vi "Add.vi"(0 "object in":refnum<class "Node.lvclass">, 2 "Value":dbl, 5 "Error In":errorcluster) -> (14 "object out":refnum<class "Node.lvclass">, 19 "Error Out":errorcluster)   [LabVIEW 2024, in "Node.lvclass"]
uses:
  Node.lvclass
  Node.lvclass/Node.ctl
  Element_interface/Element.lvclass
panel:
  # "Connector Pane"
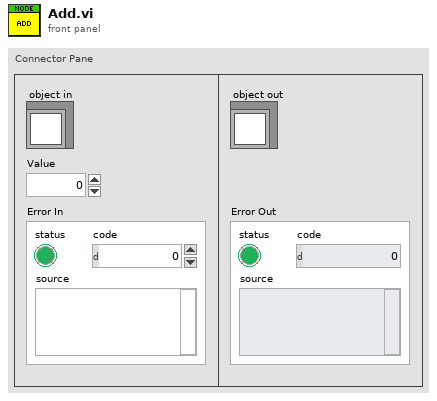
[diagram p1: front panel]
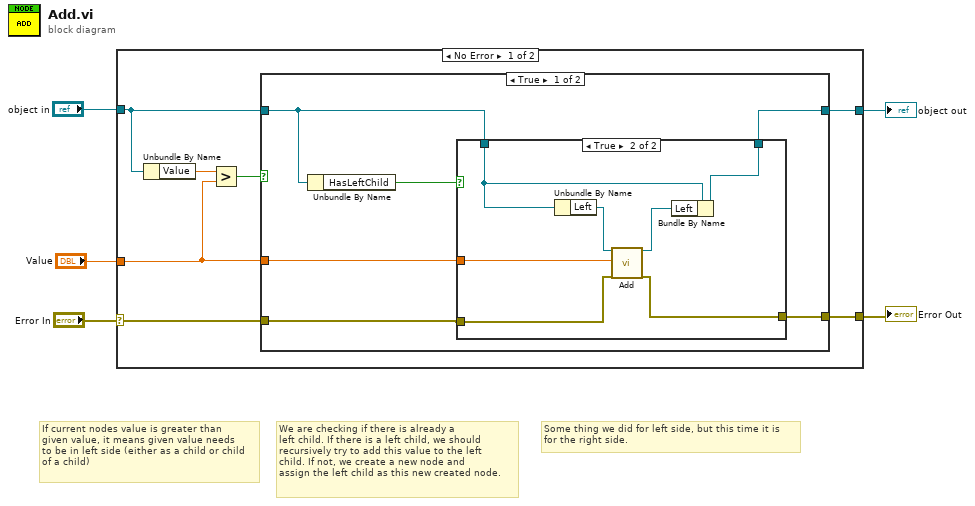
[diagram p0: block diagram]
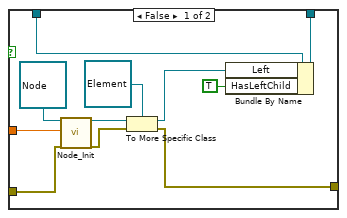
[diagram p2: hidden frame]
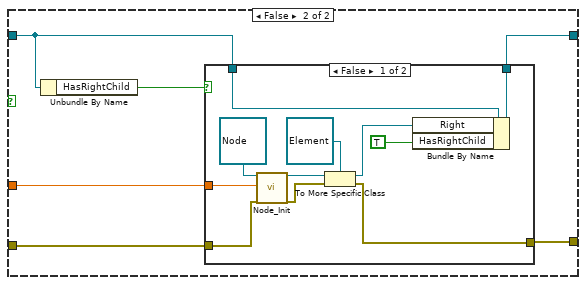
[diagram p3: hidden frame]
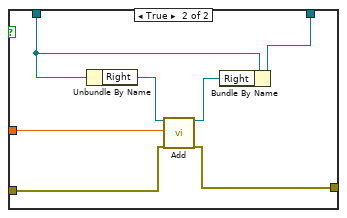
[diagram p4: hidden frame]
diagram:
  # "Some thing we did for left side, but this time it is\nfor the right side."
  # "We are checking if there is already a \nleft child. If there is a left child, we should\nrecursively try to add this value to the left\nchild. If not, we create a new node and \nassign the left child as this new created node."
  # "If current nodes value is greater than\ngiven value, it means given value needs\nto be in left side (either as a child or child\nof a child)"
  n1 = case shown="No Error" "Error In" {
    selector: "Error In" -> [w8 w62]
    tunnel: [w7 w62] -> w4
    tunnel: [w10 w61] -> w2
    tunnel: "object in" -> [w11 w61]
    tunnel: "Value" -> [w9 _]
    frame No Error {
      n2 = Unbundle By Name(w11) -> ("Value"=w6:dbl)
      n3 = Greater?(x=w6, y=w9) -> (0:w12:bool)
      n4 = case shown="True" w12 {
        tunnel: w11 -> [w15 w41]
        tunnel: [w16 w42] -> w10
        tunnel: w9 -> [w17 w37]
        tunnel: w8 -> [w14 w40]
        tunnel: [w13 w39] -> w7
        frame True {
          n5 = Unbundle By Name(w15) -> ("HasLeftChild"=w18:bool)
          n6 = case shown="True" w18 {
            tunnel: w17 -> [w28 w35]
            tunnel: w15 -> [w24 w34]
            tunnel: [w23 w33] -> w16
            tunnel: w14 -> [w20 w31]
            tunnel: [w19 w30] -> w13
            frame False {
              n7 = call "Node_Init.vi"("object in"=refnum<class "Node.lvclass"> refnum ("Node"), "Value"=w28, "Error In"=w20) -> ("object out"=w26:refnum<class "Node.lvclass">, "Error Out"=w27:errorcluster)  [unwired: 15 in]
              n8 = To More Specific Class(target class=refnum<class "Element.lvclass"> refnum ("Element"), reference=w26, error in=w27) -> (specific class reference=w22:refnum<class "Element.lvclass">, error out=w19:errorcluster)
              n9 = Bundle By Name(cluster=w24, "Left"=w22, "HasLeftChild"=TRUE) -> (w23:refnum<class "Node.lvclass">)
            }
            frame True {
              n10 = Unbundle By Name(w34) -> ("Left"=w36:refnum<class "Element.lvclass">)
              n11 = call-dynamic "Add.vi"("object in"=w36, "Value"=w35, "Error In"=w31) -> ("object out"=w32:refnum<class "Element.lvclass">, "Error Out"=w30:errorcluster)  [unwired: 15 in]
              n12 = Bundle By Name(cluster=w34, "Left"=w32) -> (w33:refnum<class "Node.lvclass">)
            }
          }
        }
        frame False {
          n13 = Unbundle By Name(w41) -> ("HasRightChild"=w38:bool)
          n14 = case shown="False" w38 {
            tunnel: w37 -> [w52 w59]
            tunnel: w41 -> [w48 w58]
            tunnel: [w47 w57] -> w42
            tunnel: w40 -> [w44 w55]
            tunnel: [w43 w54] -> w39
            frame False {
              n15 = call "Node_Init.vi"("object in"=refnum<class "Node.lvclass"> refnum ("Node"), "Value"=w52, "Error In"=w44) -> ("object out"=w50:refnum<class "Node.lvclass">, "Error Out"=w51:errorcluster)  [unwired: 15 in]
              n16 = To More Specific Class(target class=refnum<class "Element.lvclass"> refnum ("Element"), reference=w50, error in=w51) -> (specific class reference=w46:refnum<class "Element.lvclass">, error out=w43:errorcluster)
              n17 = Bundle By Name(cluster=w48, "Right"=w46, "HasRightChild"=TRUE ("HasLeftChild")) -> (w47:refnum<class "Node.lvclass">)
            }
            frame True {
              n18 = Unbundle By Name(w58) -> ("Right"=w60:refnum<class "Element.lvclass">)
              n19 = call-dynamic "Add.vi"("object in"=w60, "Value"=w59, "Error In"=w55) -> ("object out"=w56:refnum<class "Element.lvclass">, "Error Out"=w54:errorcluster)  [unwired: 15 in]
              n20 = Bundle By Name(cluster=w58, "Right"=w56) -> (w57:refnum<class "Node.lvclass">)
            }
          }
        }
      }
    }
    frame Error {
    }
  }
  "Error Out" <- w4
  "object out" <- w2
